vi "LSX Get Snapshot Par.vi"(8 "error in (no error)":errorcluster, 9 "pbAutoMode":i32, 10 "pbHigh":i32, 11 "lLSID":i32) -> (0 "error out":errorcluster, 1 "pbAutoMode out":i32, 2 "pbHigh out":i32, 3 "function return":i32)   [LabVIEW 2016, in "Tango_DLL.lvlib"]
doc: "TANGOAPI int TANGOCALL LSX_GetSnapshotPar (int lLSID, BOOL *pbHigh, BOOL *pbAutoMode);"
uses:
  Tango_DLL.lvlib
  2017/Microscope Control/Device Library/Stages/Marzhauser/SCAN IM 120 x 80/Tango DLL VIs/Tango_DLL.dll
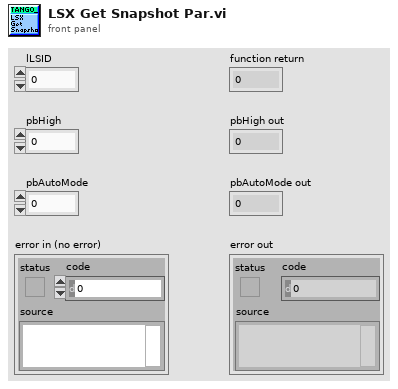
[diagram p1: front panel]
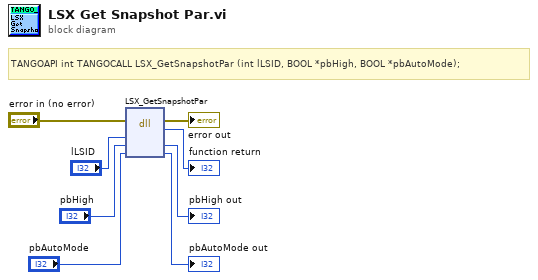
[diagram p0: block diagram]
diagram:
  # "TANGOAPI int TANGOCALL LSX_GetSnapshotPar (int lLSID, BOOL *pbHigh, BOOL *pbAutoMode);"
  n1 = dll-call lib="C:/Users/4PiSMS/Documents/Microscope Control/2017/Microscope Control/Device Library/Stages/Marzhauser/SCAN IM 120 x 80/Tango DLL VIs/Tango_DLL.*" fn="LSX_GetSnapshotPar"(error in="error in (no error)", "lLSID"="lLSID", "pbHigh"="pbHigh", "pbAutoMode"="pbAutoMode") -> (error out=→"error out":errorcluster, →"function return":i32, "pbHigh"=→"pbHigh out":i32, "pbAutoMode"=→"pbAutoMode out":i32)  [unwired: 3 in, 1 out]
